vi "Get Topic.vi"(8 "error in (no error)":errorcluster, 9 "Topic Type":variant, 10 "Topic Name":string, 11 "TopicLookupTable":refnum<data-value>) -> (0 "error out":errorcluster, 2 "Topic Enqueuer":refnum<class "Message Enqueuer.lvclass">, 3 "TopicLookupTable":refnum<data-value>)   [LabVIEW 2020, in "Mediator.lvlib" / "TopicLookupTable.lvclass"]
doc: "获取主题"
uses:
  TopicLookupTable.lvclass
  <vilib>/ActorFramework/Message Enqueuer/Message Enqueuer.lvclass
  TopicLookupTable.lvclass/TopicLookupTable.ctl
  <vilib>/ErrorRing/Error Ring.xnode
  variant-extensions/Source/VariantExtensions.lvlib
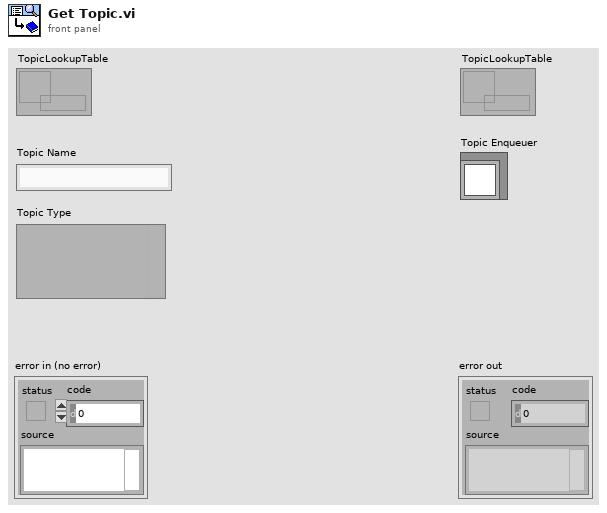
[diagram p1: front panel]
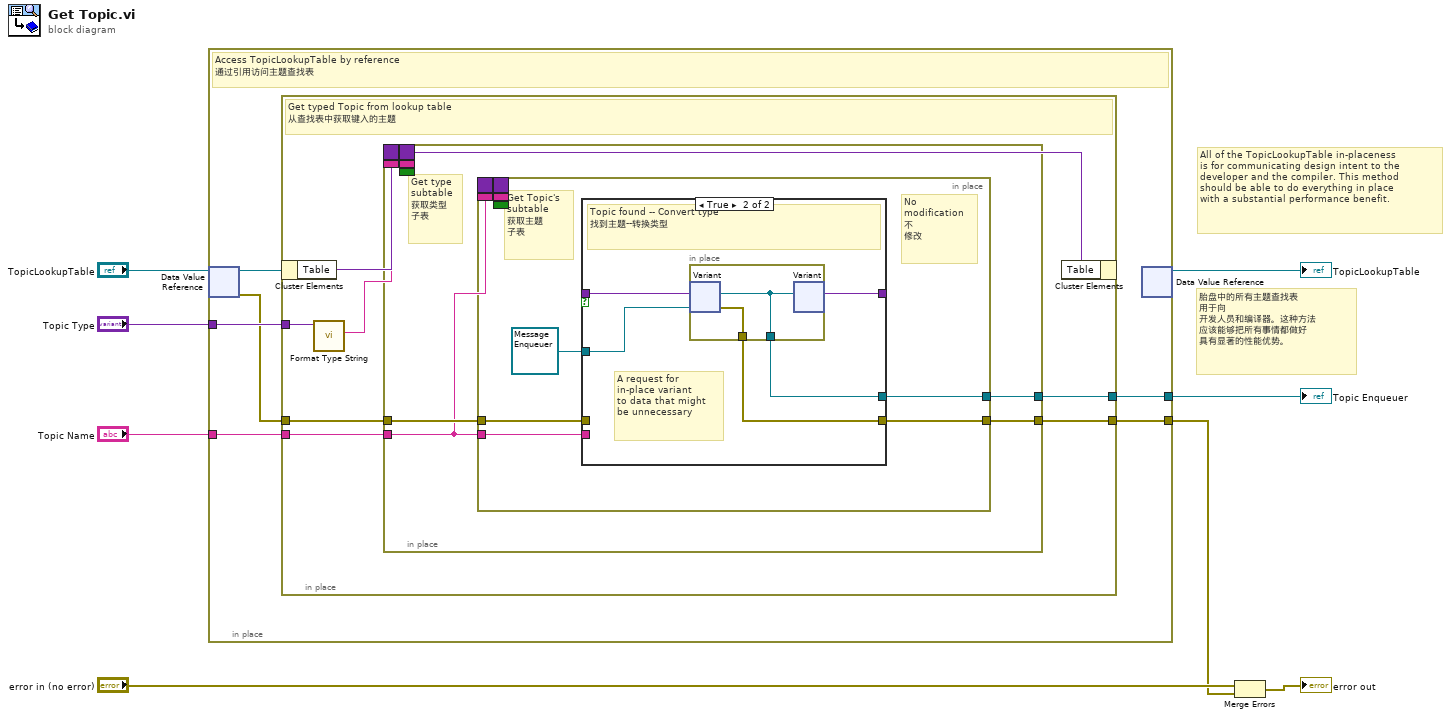
[diagram p0: block diagram]
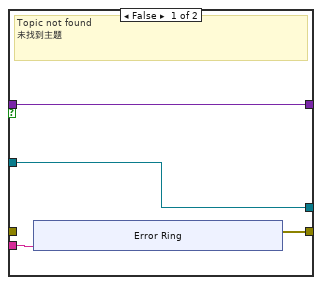
[diagram p2: hidden frame]
diagram:
  # "胎盘中的所有主题查找表\n用于向\n开发人员和编译器。这种方法\n应该能够把所有事情都做好\n具有显著的性能优势。"
  # "All of the TopicLookupTable in-placeness\nis for communicating design intent to the\ndeveloper and the compiler. This method\nshould be able to do everything in place\nwith a substantial performance benefit."
  n1 = in-place {
    in-place-border: "Topic Name" -> [w14]
    in-place-border: "Topic Type" -> [w13]
    in-place-border: [w12] -> w2
    in-place-border: [w11] -> w4
    # "Access TopicLookupTable by reference\n通过引用访问主题查找表"
    n2 = in-place-dvr #1("TopicLookupTable") -> (w10:refnum<class "TopicLookupTable.lvclass">, w9:errorcluster)
    n3 = in-place {
      in-place-border: w14 -> [w15]
      in-place-border: w13 -> [w18]
      in-place-border: [w21] -> w11
      in-place-border: [w20] -> w12
      in-place-border: w9 -> [w22]
      # "Get typed Topic from lookup table\n从查找表中获取键入的主题"
      n4 = in-place-cluster #2(w10) -> ("Table"=w19:variant)
      n5 = call "Format Type String.vi"("Data Type"=w18) -> ("Type Name"=w17:string)  [unwired: 9 in, 1 out]
      n6 = in-place {
        in-place-border: w22 -> [w24]
        in-place-border: [w28] -> w21
        in-place-border: [w25] -> w20
        in-place-border: w15 -> [w23]
        border: w19 -> [_]
        border: w17 -> [_]
        border: [_] -> w16
        border: _ -> [_]
        border: _ -> [_]
        # "Get type\nsubtable\n获取类型\n子表"
        n7 = in-place {
          in-place-border: [w36] -> w28
          border: w27 -> [_]
          border: w23 -> [_]
          border: [_] -> w26
          border: _ -> [_]
          border: _ -> [_]
          in-place-border: w23 -> [w34]
          in-place-border: [w33] -> w25
          in-place-border: w24 -> [w32]
          # "No\nmodification\n不\n修改"
          # "Get Topic's\nsubtable\n获取主题\n子表"
          n8 = case shown="True" w35 {
            tunnel: [w37 w46] -> w36
            tunnel: w34 -> [w40 _]
            tunnel: [w39 w48] -> w33
            tunnel: w32 -> [_ _]
            tunnel: w31 -> [w38 w50]
            tunnel: [w38 w49] -> w30
            tunnel: refnum<class "Message Enqueuer.lvclass"> refnum ("Self Enqueuer") -> [w37 w47]
            frame False {
              # "Topic not found\n未找到主题"
              n9 = xnode "Error Ring"("parameter 0"=w40) -> ("error out"=w39:errorcluster)
            }
            frame True {
              # "A request for\nin-place variant\nto data that might\nbe unnecessary"
              # "Topic found -- Convert type\n找到主题--转换类型"
              n10 = in-place {
                in-place-border: [w52] -> w46
                in-place-border: [w51] -> w48
                n11 = in-place-variant #3(w50, w47) -> (w52:refnum<class "Message Enqueuer.lvclass">, w51:errorcluster)
                n12 = in-place-variant #3(w52) -> (w49:variant)  [unwired: 1 out]
              }
            }
          }
        }
      }
      n13 = in-place-cluster #2("Table"=w16) -> ()  [unwired: 1 out]
    }
    n14 = in-place-dvr #1() -> (→"TopicLookupTable":refnum<data-value>)  [unwired: 1 in, 1 out]
  }
  "Topic Enqueuer" <- w4
  n15 = Merge Errors("error in (no error)", w2) -> (→"error out":errorcluster)
